vi "calculate_XOR.vi"(1 "Divisor":u8[](array[numeric]), 2 "Initial Poly":u8[](array[numeric])) -> (0 "Array":u8[](array[numeric]))   [LabVIEW 2022 SP3]
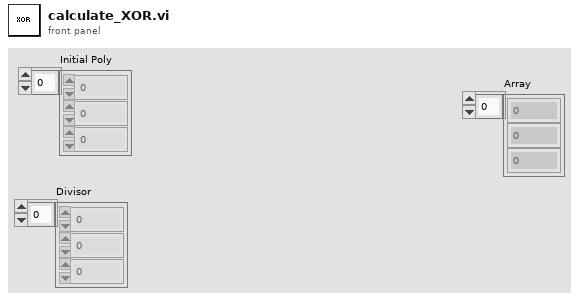
[diagram p1: front panel]
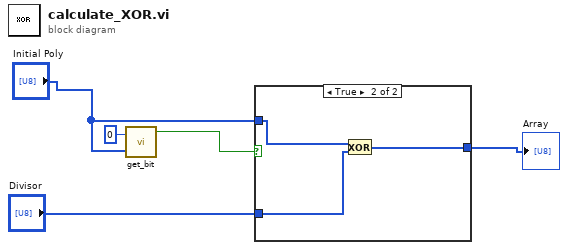
[diagram p0: block diagram]
diagram:
  n1 = call "get_bit.vi"("Position"=u16 0, "INFO"="Initial Poly") -> ("Bit_Value"=w4:bool)  [unwired: 2 out]
  n2 = case shown="True" w4 {
    tunnel: "Initial Poly" -> [w6 w9]
    tunnel: "Divisor" -> [_ w8]
    tunnel: [w6 w7] -> w1
    frame False {
    }
    frame True {
      n3 = Exclusive Or(1:w8, 2:w9) -> (0:w7:u8[])
    }
  }
  "Array" <- w1
